vi "Reset device names.vi"(6 "Defer restart? (true)":bool=TRUE, 8 "error in (no error)":errorcluster, 11 "RT Management in":refnum<class "RT Management.lvclass">) -> (0 "error out":errorcluster, 3 "RT Management out":refnum<class "RT Management.lvclass">)   [LabVIEW 2015, in "RT Management.lvlib" / "RT Management.lvclass"]
doc: "Resets all device names back to \"PXI1Slot<device slot>\". The slot is hard-coded due to the current inability of the System Configuration API to renumber a chassis (coming in 2015). Supported exports: daqmx, ni-visa. Unsupported experts: ni-rio (coming in 2014)."
uses:
  RT Management.lvclass
  RT Management.lvclass/RT Management.ctl
  Get SysCfg Session.vi
  <vilib>/nisyscfg/Find Hardware.vi
  <vilib>/nisyscfg/Close (Filter).vi
  <vilib>/nisyscfg/Close (Hardware).vi
  <vilib>/nisyscfg/nisyscfg.lvlib
  <resource>/objmgr/nisysapi.rc
  <resource>/objmgr/niflexriosae.rc
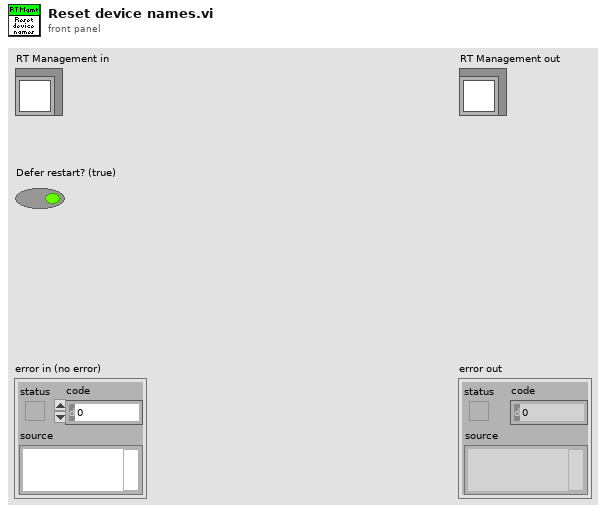
[diagram p1: front panel]
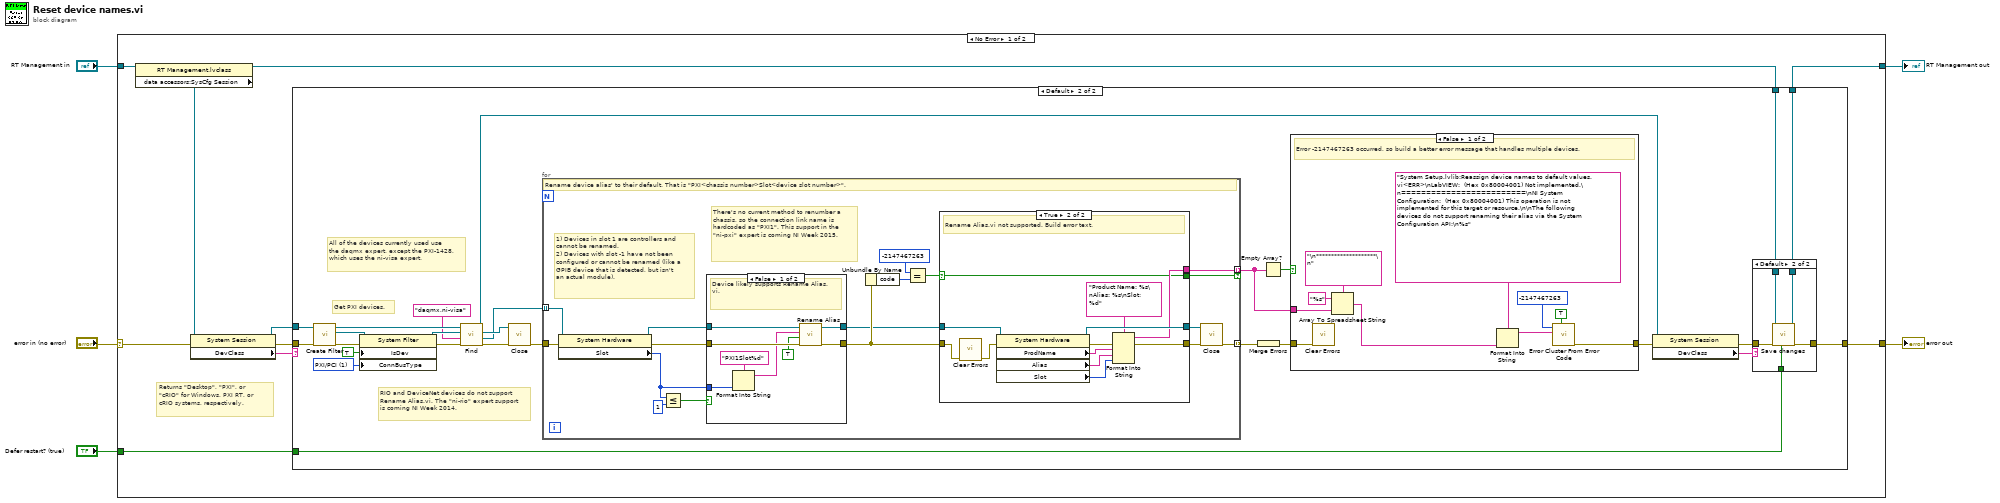
[diagram p0: block diagram]
diagram:
  n1 = case shown="No Error" "error in (no error)" {
    selector: "error in (no error)" -> [w10 w104]
    tunnel: [w7 w104] -> w3
    tunnel: "RT Management in" -> [w12 w103]
    tunnel: [w8 w103] -> w2
    tunnel: "Defer restart? (true)" -> [w6 _]
    frame No Error {
      # "Returns \"Desktop\", \"PXI\", or \"cRIO\" for Windows, PXI RT, or cRIO systems, respectively."
      n2 = property class="RT Management.lvclass"(reference=w12) -> (reference out=w9:refnum<class "RT Management.lvclass">, "data accessors:SysCfg Session"=w11:refnum<k21>)  [unwired: 1 in, 1 out]
      n3 = property class="System Session"(reference=w11, error in=w10) -> (reference out=w14:refnum<k21>, error out=w15:errorcluster, "DevClass"=w13:string)
      n4 = case shown="Default" w13 {
        tunnel: [w17 w32] -> w7
        tunnel: w15 -> [w17 w22]
        tunnel: w14 -> [_ w21]
        tunnel: w9 -> [w16 w20]
        tunnel: [w16 w19] -> w8
        tunnel: w6 -> [_ w18]
        frame "cRIO" {
        }
        frame Default {
          w33 = u32 1 items=["BuiltIn/System", "PXI/PCI", "USB", "GPIB", "VXI", "Serial", "TCP/IP", "cRIO", "SCXI", "cDAQ", "SwitchBlock", "SCC"] ("Devices & Chassis:Connects To Bus Type")
          # "All of the devices currently used use the daqmx expert, except the PXI-1428, which uses the ni-visa expert."
          # "RIO and DeviceNet devices do not support Rename Alias.vi. The \"ni-rio\" expert support is coming NI Week 2014."
          # "Get PXI devices."
          n5 = call <vilib>:"Create Filter.vi"("error in (no error)"=w22, "Session in"=w21) -> ("error out"=w43:errorcluster, "Filter out"=w41:refnum<k20>, "Session out"=w38:refnum<k21>)  [unwired: 7 in]
          n6 = property class="System Filter"(reference=w41, error in=w43, "IsDev"=TRUE ("Is Chassis"), "ConnBusType"=w33) -> (reference out=w39:refnum<k20>, error out=w40:errorcluster)
          n7 = call-poly <vilib>:"Find.vi"("error in (no error)"=w40, "Experts"="daqmx,ni-visa" ("experts"), "Filter in"=w39, "Session in"=w38) -> ("error out"=w37:errorcluster, "Resources out"=w35:refnum<k20>[], "Filter out"=w36:refnum<k20>, "Session out"=w24:refnum<k21>)  [unwired: 4 in]
          n8 = call-poly <vilib>:"Close.vi"("error in (no error)"=w37, "Filter in"=w36) -> ("error out"=w34:errorcluster)  [unwired: 9 in]
          n9 = for {
            tunnel: w34 -> [w77]
            tunnel: w35 -> [w78] mode=indexing
            tunnel: [w65] -> w28 mode=indexing if=w64
            tunnel: [w63] -> w31 mode=indexing
            # "There's no current method to renumber a chassis, so the connection link name is hardcoded as \"PXI1\". This support in the \"ni-pxi\" expert is coming NI Week 2015."
            # "1) Devices in slot 1 are controllers and cannot be renamed.\n2) Devices with slot -1 have not been configured or cannot be renamed (like a GPIB device that is detected, but isn't an actual module)."
            # "Rename device alias' to their default. That is \"PXI<chassis number>Slot<device slot number>\"."
            n10 = property class="System Hardware"(reference=w78, error in=w77) -> (reference out=w75:refnum<k20>, error out=w76:errorcluster, "Slot"=w73:i32)
            n11 = Less Or Equal?(x=w73, y=1) -> (x <= y?=w62:bool)
            n12 = case shown="False" w62 {
              tunnel: w76 -> [w100 w101]
              tunnel: w75 -> [w99 w102]
              tunnel: [w97 w102] -> w68
              tunnel: [w96 w101] -> w69
              tunnel: w73 -> [w94 _]
              frame False {
                # "Device likely supports Rename Alias.vi."
                n13 = Format Into String(format string="PXI1Slot%d", w94) -> (resulting string=w93:string)  [unwired: 2 in, 1 out]
                n14 = call <vilib>:"Rename Alias.vi"("error in (no error)"=w100, "Overwrite Conflict (F)"=TRUE ("overwrite (F)"), "New Name"=w93, "Resource in"=w99) -> ("error out"=w96:errorcluster, "Resource out"=w97:refnum<k20>)  [unwired: 4 in, 2 out]
              }
              frame True {
                # "Device doesn't support Rename Alias.vi."
              }
            }
            n15 = Unbundle By Name(w69) -> ("code"=w72:i32)
            n16 = Equal?(x=-2147467263, y=w72) -> (x = y?=w70:bool)
            n17 = case shown="True" w70 {
              selector: w70 -> [_ w85]
              tunnel: w69 -> [w80 w82]
              tunnel: w68 -> [w79 w92]
              tunnel: [w80 w83] -> w67
              tunnel: [w79 w91] -> w66
              tunnel: [_ w86] -> w65
              tunnel: [_ w85] -> w64
              frame False {
                # "Something else."
              }
              frame True {
                # "Rename Alias.vi not supported. Build error text."
                n18 = call <vilib>:"Clear Errors.vi"("error in (no error)"=w82) -> ("error out"=w81:errorcluster)  [unwired: 5 in, 1 out]
                n19 = property class="System Hardware"(reference=w92, error in=w81) -> (reference out=w91:refnum<k20>, error out=w84:errorcluster, "ProdName"=w90:string, "Alias"=w89:string, "Slot"=w88:i32)
                n20 = Format Into String(format string="Product Name: %s\nAlias: %s\nSlot: %d", error in=w84, w90, w89, w88) -> (resulting string=w86:string, error out=w83:errorcluster)  [unwired: 1 in]
              }
            }
            n21 = call-poly <vilib>:"Close.vi"("error in (no error)"=w67, "Resource in"=w66) -> ("error out"=w63:errorcluster)  [unwired: 9 in]
          }
          n22 = Merge Errors(w31) -> (w30:errorcluster)
          n23 = Empty Array?(array=w28) -> (empty?=w29:bool)
          n24 = case shown="False" w29 {
            tunnel: w30 -> [w59 w61]
            tunnel: w28 -> [w57 _]
            tunnel: [w52 w61] -> w26
            frame False {
              # "Error -2147467263 occurred, so build a better error message that handles multiple devices."
              n25 = call <vilib>:"Clear Errors.vi"("error in (no error)"=w59) -> ()  [unwired: 5 in, 2 out]
              n26 = Array To Spreadsheet String(delimiter (Tab)="\n********************\n", array=w57, 3:"%s" ("format string")) -> (spreadsheet string=w55:string)
              n27 = Format Into String(format string="System Setup.lvlib:Reassign device names to default values.vi<ERR>\nLabVIEW:  (Hex 0x80004001) Not implemented.\n=========================\nNI System Configuration:  (Hex 0x80004001) This operation is not implemented for this target or resource.\n\nThe following devices do not support renaming their alias via the System Configuration API:\n%s", w55) -> (resulting string=w53:string)  [unwired: 2 in, 1 out]
              n28 = call <vilib>:"Error Cluster From Error Code.vi"("show call chain? (False)"=TRUE, "error message (\"\")"=w53, "error code (0)"=-2147467263 ("x")) -> ("error out"=w52:errorcluster)  [unwired: 6 in]
            }
            frame True {
              # "Something else."
            }
          }
          n29 = property class="System Session"(reference=w24, error in=w26) -> (error out=w25:errorcluster, "DevClass"=w23:string)  [unwired: 1 out]
          n30 = case shown="Default" w23 {
            tunnel: [w45 w49] -> w32
            tunnel: w25 -> [w45 w50]
            tunnel: w20 -> [w44 w48]
            tunnel: [w44 w47] -> w19
            tunnel: w18 -> [_ w46]
            frame "Desktop" {
            }
            frame Default {
              n31 = call "Save changes.vi"("Defer restart? (true)"=w46, "error in (no error)"=w50, "RT Management in"=w48) -> ("error out"=w49:errorcluster, "RT Management out"=w47:refnum<class "RT Management.lvclass">)  [unwired: 7 in]
            }
          }
        }
      }
    }
    frame Error {
    }
  }
  "error out" <- w3
  "RT Management out" <- w2
